vi "Test_logEvent_settingsApplied.vi"(8 "error in (no error)":errorcluster, 11 "logevent_settingsApplied_Ctl":T1={"TestID"=0, "private_revCode"="        ", "private_sndStamp"=0.0, "private_rcvStamp"=0.0, "private_seqNum"=0, "private_identity"="", "private_origin"=0, "private_host"=0, "settingsVersion"="                                                                                                                                                                                                                                                                ", "otherSettingsEvents"="", "priority"=0}) -> (0 "error out":errorcluster, 2 "function return":i32, 3 "logevent_settingsApplied_Ctl out":T1={"TestID"=0, "private_revCode"="        ", "private_sndStamp"=0.0, "private_rcvStamp"=0.0, "private_seqNum"=0, "private_identity"="", "private_origin"=0, "private_host"=0, "settingsVersion"="                                                                                                                                                                                                                                                                ", "otherSettingsEvents"="", "priority"=0})   [LabVIEW 2018, in "SALLV_Test.lvlib"]
doc: "int Test_shm_logEvent_settingsAppliedLV(Test_logevent_settingsAppliedLV *logevent_settingsApplied_Ctl );"
uses:
  DataTypes/logevent_settingsApplied.ctl
  SALLV_Test.lvlib
  SALLV_Test.so
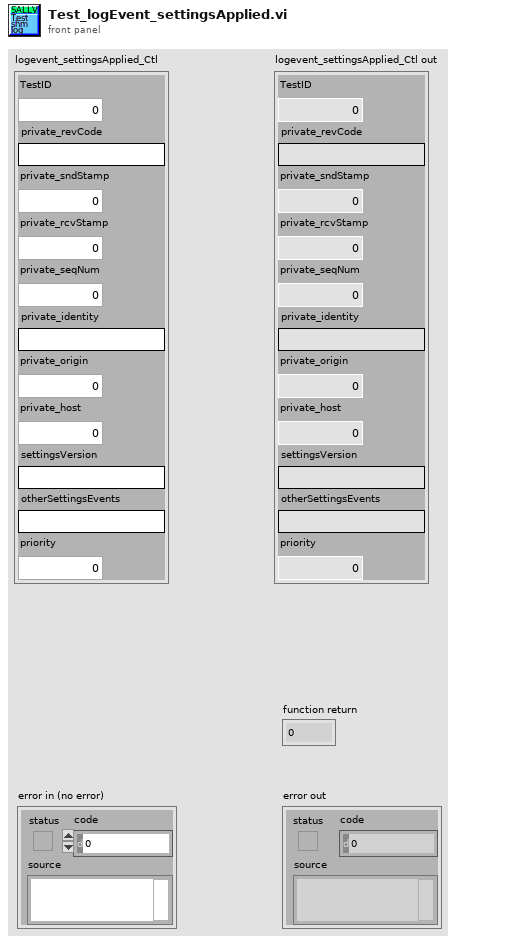
[diagram p1: front panel]
types:
  T1 = typedef "SALLV_Test.lvlib/logevent_settingsApplied.ctl" = cluster{"TestID":i32, "private_revCode":string, "private_sndStamp":dbl, "private_rcvStamp":dbl, "private_seqNum":i32, "private_identity":string, "private_origin":i32, "private_host":i32, "settingsVersion":string, "otherSettingsEvents":string, "priority":i32}
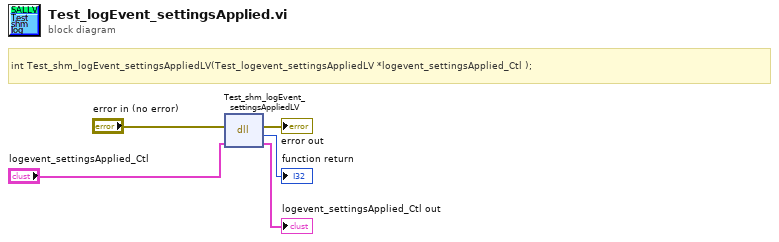
[diagram p0: block diagram]
diagram:
  # "int Test_shm_logEvent_settingsAppliedLV(Test_logevent_settingsAppliedLV *logevent_settingsApplied_Ctl );"
  n1 = dll-call lib="home/ttsai/Documents/github/ts_SALLabVIEW/testPerfTemp/TestData/SALLV_Test.*" fn="Test_shm_logEvent_settingsAppliedLV"(error in="error in (no error)", "logevent_settingsApplied_Ctl"="logevent_settingsApplied_Ctl") -> (error out=→"error out":errorcluster, →"function return":i32, "logevent_settingsApplied_Ctl"=→"logevent_settingsApplied_Ctl out":T1)  [unwired: 2 in, 1 out]
